vi "Get Item Names in MCListbox.vi"(8 "error in":errorcluster, 10 "Label":string, 11 "Class in":refnum<class>) -> (0 "error out":errorcluster, 2 "Item Names":string[][](array[string]), 3 "Class out":refnum<class>)   [LabVIEW 2023, in "Label-Driven UI.lvlib"]
uses:
  Label-Driven UI.lvlib
  ace85fde-b992-4b3d-a1e9-8eef8c0f64fe.vi
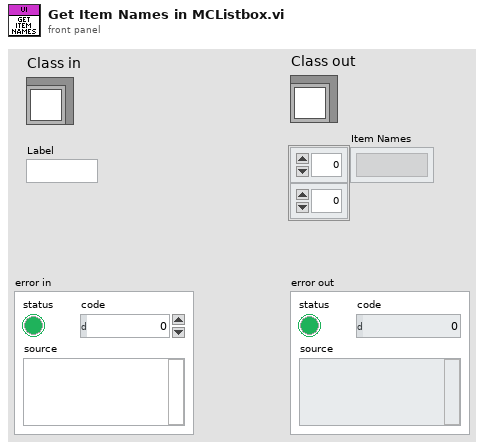
[diagram p1: front panel]
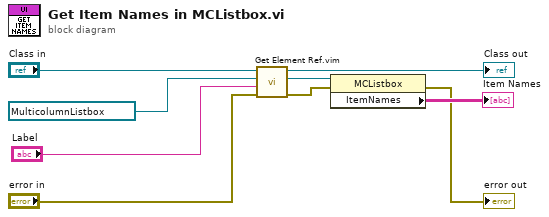
[diagram p0: block diagram]
diagram:
  n1 = call "Get Element Ref.vim"("error in"="error in", "Label"="Label", "Ref Type"=refnum<vi> refnum, "Class in"="Class in") -> ("error out"=w3:errorcluster, "Element Ref"=w4:refnum<vi>, "Class out"=→"Class out":refnum<class>)  [unwired: 5 in]
  n2 = property class="MCListbox"(reference=w4, error in=w3) -> (error out=→"error out":errorcluster, "ItemNames"=→"Item Names":string[][])  [unwired: 1 out]
